vi "Check parts acceptable - baselayer.vi"(8 "error in (no error)":errorcluster, 9 "Baselayer IDs":string[](array[string]), 10 "DB out base":string[][](array[string]), 11 "Database Entry in":refnum<class "Database Entry.lvclass">) -> (0 "error out":errorcluster, 1 "Thickness out":string[](array[string]), 2 "Replace parts out":bool, 3 "Database Entry out":refnum<class "Database Entry.lvclass">, 4 "Abort?":bool)   [LabVIEW 2021, in "Database Entry.lvclass"]
uses:
  Database Entry.lvclass
  Database Entry.lvclass/Database Entry.ctl
  Components/Stack/Stack.lvclass
panel:
  in  "Replace parts base":bool
  in  "Thickness column options to use for assembly":u16(ring) items=["avg_thickness", "max_thickness"]
  in  "Are these parts satisfactory?":bool
  in  "Abort":bool
  in  "Submit":bool
  in  "Proposed thickness for assembly dispense":string[](array[string])
  in  "Database out - baselayer":i32[](listbox)
  # "Modify thickness values manually, if needed"
  # "(If parts are satisfactory, this assembly run will be written into Postgres.)"
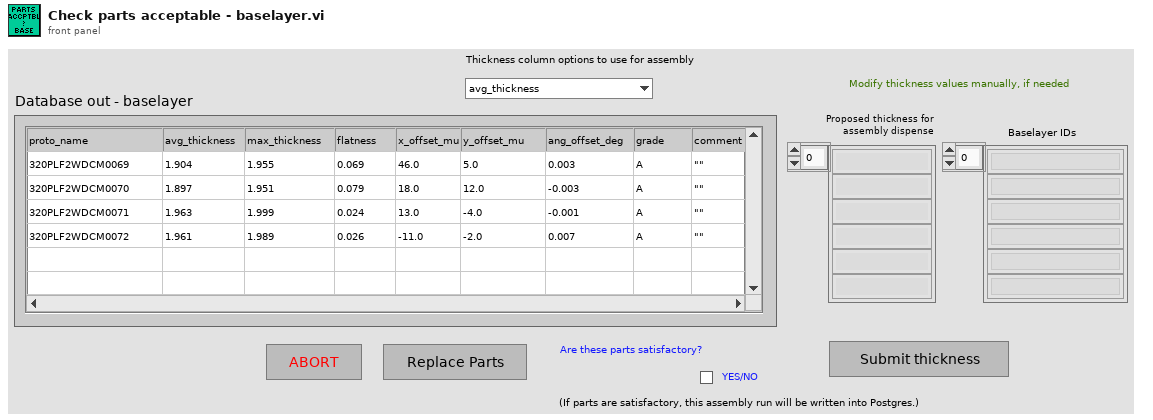
[diagram p1: front panel]
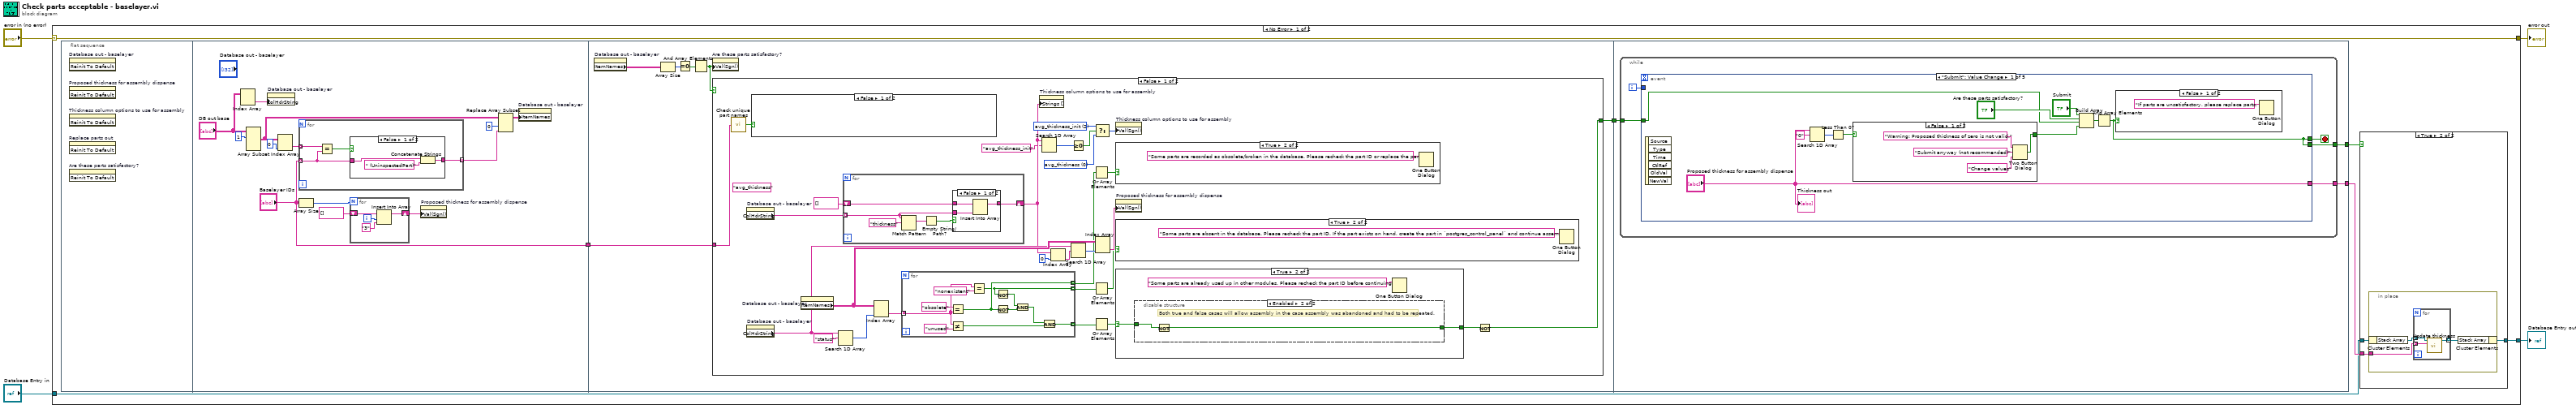
[diagram p0: block diagram]
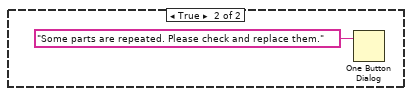
[diagram p5: hidden frame]
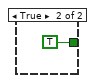
[diagram p10: hidden frame]
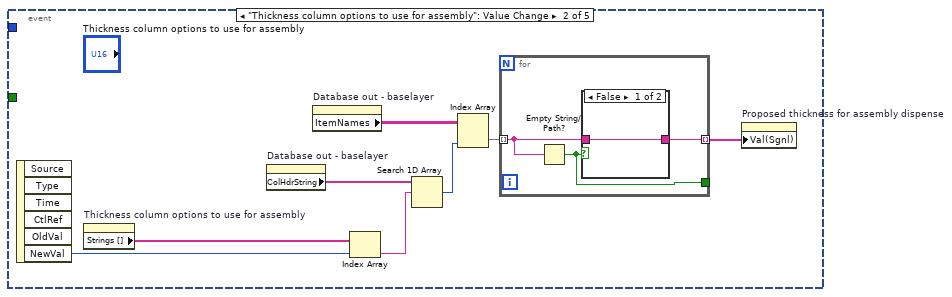
[diagram p13: hidden frame]
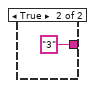
[diagram p14: hidden frame]
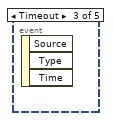
[diagram p15: hidden frame]
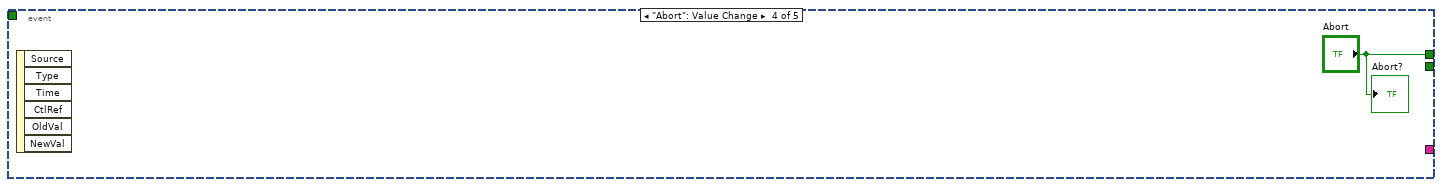
[diagram p16: hidden frame]
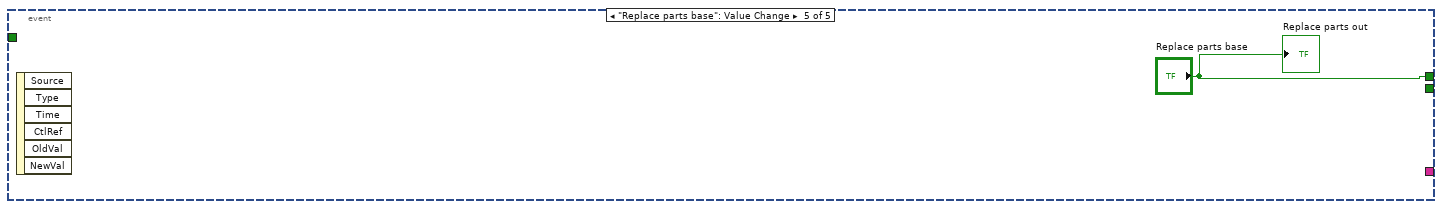
[diagram p17: hidden frame]
diagram:
  n1 = case shown="No Error" "error in (no error)" {
    selector: "error in (no error)" -> [w11 w153]
    tunnel: [w11 w153] -> w3
    tunnel: [w7 w152] -> w1
    tunnel: "Database Entry in" -> [w8 w152]
    frame No Error {
      n2 = flat-sequence {
        tunnel: ["Baselayer IDs"] -> w6
        tunnel: w6 -> [w47]
        tunnel: [w48] -> w5
        tunnel: [w115] -> w10
        tunnel: [w114] -> w9
        tunnel: w5 -> [w113]
        frame #0 {
          n3 = invoke on="Database out - baselayer" class="MCListbox (strict)" method="Reinit To Default"() -> ()  [unwired: 3 in, 3 out]
          n4 = invoke on="Proposed thickness for assembly dispense" class="Arr (strict)" method="Reinit To Default"() -> ()  [unwired: 3 in, 3 out]
          n5 = invoke on="Thickness column options to use for assembly" class="Ring (strict)" method="Reinit To Default"() -> ()  [unwired: 3 in, 3 out]
          n6 = invoke on="Replace parts out" class="Bool (strict)" method="Reinit To Default"() -> ()  [unwired: 3 in, 3 out]
          n7 = invoke on="Are these parts satisfactory?" class="Bool (strict)" method="Reinit To Default"() -> ()  [unwired: 3 in, 3 out]
        }
        frame #1 {
          n8 = Index Array(array="DB out base") -> (element=w27:string[])  [unwired: 2 in]
          n9 = Array Subset(array="DB out base", index (row)=1 ("index")) -> (w31:string[][])  [unwired: 3 in]
          n10 = property on="Database out - baselayer" class="MCListbox (strict)"("ColHdrString"=w27) -> ()  [unwired: 2 in, 2 out]
          n11 = Index Array(array=w31, index (col)=0 ("disabled index (col)")) -> (element=w32:string[])  [unwired: 1 in]
          n12 = for {
            tunnel: w32 -> [w41] mode=indexing
            tunnel: "Baselayer IDs" -> [w39] mode=indexing
            tunnel: [w40] -> w29 mode=indexing
            n13 = Equal?(x=w41, y=w39) -> (x = y?=w42:bool)
            n14 = case shown="False" w42 {
              tunnel: w39 -> [w45 w46]
              tunnel: [w43 w46] -> w40
              frame False {
                n15 = Concatenate Strings(w45, " (UninspectedPart)" ("string")) -> (w43:string)
              }
              frame True {
              }
            }
          }
          n16 = Array Size(array="Baselayer IDs") -> (size(s)=w25:i32)
          n17 = for {
            N: w25 -> [_]
            shift-right: [w35] -> w23
            shift-left: string[] [] -> [w38]
            i -> [w36]
            n18 = Insert Into Array(array=w38, index=w36, new element="3" ("new element/subarray")) -> (w35:string[])
          }
          n19 = property on="Proposed thickness for assembly dispense" class="Arr (strict)"("Val(Sgnl)"=w23) -> ()  [unwired: 2 in, 2 out]
          n20 = Replace Array Subset(array=w31, new element=w29, index (col)=0 ("disabled index (col)")) -> (w26:string[][])  [unwired: 1 in]
          n21 = property on="Database out - baselayer" class="MCListbox (strict)"("ItemNames"=w26) -> ()  [unwired: 2 in, 2 out]
        }
        frame #2 {
          n22 = property on="Database out - baselayer" class="MCListbox (strict)"() -> ("ItemNames"=w50:string[][])  [unwired: 2 in, 2 out]
          n23 = Array Size(array=w50) -> (size(s)=w51:i32[])
          n24 = Equal To 0?(x=w51) -> (x = 0?=w52:bool[])
          n25 = And Array Elements(Boolean array=w52) -> (logical AND=w49:bool)
          n26 = property on="Are these parts satisfactory?" class="Bool (strict)"("Val(Sgnl)"=w49) -> ()  [unwired: 2 in, 2 out]
          n27 = case shown="False" w49 {
            tunnel: w47 -> [w69 _]
            tunnel: [w66 TRUE] -> w48
            frame False {
              w53 = u16 0 items=["avg_thickness", "max_thickness", "avg_thickness_init", "max_thickness_init"] ("Thickness column options to use for assembly")
              w55 = u16 2 items=["avg_thickness", "max_thickness", "avg_thickness_init", "max_thickness_init"] ("Thickness column options to use for assembly")
              (unwired) "avg_thickness" ("f")
              n28 = call "Check unique part names.vi"("Part IDs"=w69) -> ("Parts repeated"=w68:bool)
              n29 = property on="Database out - baselayer" class="MCListbox (strict)"() -> ("ColHdrString"=w79:string[])  [unwired: 2 in, 2 out]
              n30 = property on="Database out - baselayer" class="MCListbox (strict)"() -> ("ColHdrString"=w73:string[])  [unwired: 2 in, 2 out]
              n31 = case shown="False" w68 {
                frame False {
                }
                frame True {
                  n32 = One Button Dialog(message="Some parts are repeated. Please check and replace them.") -> ()  [unwired: 1 in, 1 out]
                }
              }
              n33 = property on="Database out - baselayer" class="MCListbox (strict)"() -> ("ItemNames"=w74:string[][])  [unwired: 2 in, 2 out]
              n34 = Search 1D Array(1D array=w73, element="status") -> (index of element=w71:i32)  [unwired: 1 in]
              n35 = for {
                tunnel: w79 -> [w104] mode=indexing
                shift-right: [w103] -> w59
                shift-left: string[] [] -> [w102]
                n36 = Match Pattern(string=w104, regular expression="thickness") -> (match substring=w106:string)  [unwired: 1 in, 3 out]
                n37 = Empty String/Path?(string/path=w106) -> (empty?=w105:bool)
                n38 = case shown="False" w105 {
                  tunnel: [w108 w111] -> w103
                  tunnel: w104 -> [w109 _]
                  tunnel: w102 -> [w110 w111]
                  frame False {
                    n39 = Insert Into Array(array=w110, new element=w109) -> (w108:string[])  [unwired: 1 in]
                  }
                  frame True {
                  }
                }
              }
              n40 = Index Array(array=w74, index (col)=w71) -> (element=w65:string[])  [unwired: 1 in]
              n41 = for {
                tunnel: w65 -> [w91] mode=indexing
                tunnel: [w98] -> w63 mode=indexing
                tunnel: [w95] -> w64 mode=indexing
                tunnel: [w97] -> w61 mode=indexing
                n42 = Equal?(x="obsolete" ("y"), y=w91) -> (x = y?=w97:bool)
                n43 = Not Equal?(x=w91, y="unused") -> (x != y?=w100:bool)
                n44 = Equal?(x=w91, y="nonexistent") -> (x = y?=w95:bool)
                n45 = Not(x=w95) -> (.not. x?=w94:bool)
                n46 = Not(x=w97) -> (.not. x?=w96:bool)
                n47 = And(x=w94, y=w96) -> (x .and. y?=w93:bool)
                n48 = And(x=w93, y=w100) -> (x .and. y?=w98:bool)
              }
              n49 = property on="Thickness column options to use for assembly" class="Ring (strict)"("Strings []"=w59) -> ()  [unwired: 2 in, 2 out]
              n50 = Search 1D Array(1D array=w59, element="avg_thickness_init") -> (index of element=w58:i32)  [unwired: 1 in]
              n51 = Index Array(array=w59, index=0) -> (element=w80:string)
              n52 = Greater Or Equal To 0?(x=w58) -> (x >= 0?=w57:bool)
              n53 = Search 1D Array(1D array=w73, element=w80) -> (index of element=w76:i32)  [unwired: 1 in]
              n54 = Or Array Elements(Boolean array=w61) -> (logical OR=w60:bool)
              n55 = Or Array Elements(Boolean array=w64) -> (logical OR=w70:bool)
              n56 = Or Array Elements(Boolean array=w63) -> (logical OR=w62:bool)
              n57 = Select(t=w55, s=w57, f=w53) -> (s? t:f=w54:u16)
              n58 = Index Array(array=w74, index (col)=w76) -> (element=w75:string[])  [unwired: 1 in]
              n59 = property on="Thickness column options to use for assembly" class="Ring (strict)"("Val(Sgnl)"=w54) -> ()  [unwired: 2 in, 2 out]
              n60 = case shown="True" w60 {
                frame False {
                }
                frame True {
                  n61 = One Button Dialog(message="Some parts are recorded as obsolete/broken in the database. Please recheck the part ID or replace the part.") -> ()  [unwired: 1 in, 1 out]
                }
              }
              n62 = property on="Proposed thickness for assembly dispense" class="Arr (strict)"("Val(Sgnl)"=w75) -> ()  [unwired: 2 in, 2 out]
              n63 = case shown="True" w70 {
                frame False {
                }
                frame True {
                  n64 = One Button Dialog(message="Some parts are absent in the database. Please recheck the part ID. If the part exists on hand, create the part in `postgres_control_panel` and continue assembly. ") -> ()  [unwired: 1 in, 1 out]
                }
              }
              n65 = case shown="True" w62 {
                selector: w62 -> [w83 w85]
                tunnel: [w83 w84] -> w67
                frame False {
                }
                frame True {
                  n66 = disable-structure shown="Enabled" {
                    disable-tunnel: w85 -> [w87 w89]
                    disable-tunnel: [w87 w88] -> w84
                    frame Disabled {
                    }
                    frame Enabled {
                      # "Both true and false cases will allow assembly in the case assembly was abandoned and had to be repeated."
                      n67 = Not(x=w89) -> (.not. x?=w88:bool)
                    }
                  }
                  n68 = One Button Dialog(message="Some parts are already used up in other modules. Please recheck the part ID before continuing.") -> ()  [unwired: 1 in, 1 out]
                }
              }
              n69 = Not(x=w67) -> (.not. x?=w66:bool)
            }
            frame True {
            }
          }
        }
        frame #3 {
          n70 = while {
            tunnel: [w118] -> w115
            tunnel: [w120] -> w114
            tunnel: w113 -> [w117]
            i -> [w116]
            stop <- w119 stop-if-true
            n71 = event shown="[0] \"Submit\": Value Change" {
              selector: _ -> [_ _ _ _ _]
              dyn-events: _ -> [_ _ _ _ _]
              timeout: _ -> [_ _ _ _ _]
              tunnel: [w126 _ _ "Abort" "Replace parts base"] -> w119
              tunnel: ["Proposed thickness for assembly dispense" _ _ _ _] -> w120
              tunnel: [w126 _ _ _ _] -> w118
              tunnel: w117 -> [w127 _ _ _ _]
              tunnel: w116 -> [_ _ _ _ _]
              event "Submit": Value Change {
                n72 = event-data() -> ()  [unwired: 1 in, 6 out]
                n73 = Search 1D Array(1D array="Proposed thickness for assembly dispense", element="0") -> (index of element=w123:i32)  [unwired: 1 in]
                n74 = Less Than 0?(x=w123) -> (x < 0?=w122:bool)
                n75 = case shown="False" w122 {
                  selector: w122 -> [_ w135]
                  tunnel: [w134 w135] -> w121
                  frame False {
                    n76 = Two Button Dialog(message="Warning: Proposed thickness of zero is not valid.", 1:"Change values" ("T button name (\"OK\")"), 2:"Submit anyway (not recommended)" ("F button name (\"Cancel\")")) -> (T button?=w134:bool)
                  }
                  frame True {
                  }
                }
                n77 = Build Array("Submit", "Are these parts satisfactory?", w127, w121) -> (w130:bool[])
                n78 = And Array Elements(Boolean array=w130) -> (logical AND=w126:bool)
                n79 = case shown="False" w126 {
                  frame False {
                    n80 = One Button Dialog(message="If parts are unsatisfactory, please replace parts. ") -> ()  [unwired: 1 in, 1 out]
                  }
                  frame True {
                  }
                }
                "Thickness out" <- "Proposed thickness for assembly dispense"
              }
              event "Thickness column options to use for assembly": Value Change {
                n81 = event-data() -> ("NewVal"=w143:u16)  [unwired: 1 in, 5 out]
                n82 = property on="Thickness column options to use for assembly" class="Ring (strict)"() -> ("Strings []"=w144:string[])  [unwired: 2 in, 2 out]
                n83 = property on="Database out - baselayer" class="MCListbox (strict)"() -> ("ColHdrString"=w140:string[])  [unwired: 2 in, 2 out]
                n84 = property on="Database out - baselayer" class="MCListbox (strict)"() -> ("ItemNames"=w141:string[][])  [unwired: 2 in, 2 out]
                n85 = Index Array(array=w144, index=w143) -> (element=w142:string)
                n86 = Search 1D Array(1D array=w140, element=w142) -> (index of element=w139:i32)  [unwired: 1 in]
                n87 = Index Array(array=w141, index (col)=w139) -> (element=w138:string[])  [unwired: 1 in]
                n88 = for {
                  tunnel: w138 -> [w147] mode=indexing
                  tunnel: [w146] -> w137 mode=indexing
                  tunnel: [w145] -> _
                  n89 = Empty String/Path?(string/path=w147) -> (empty?=w145:bool)
                  n90 = case shown="False" w145 {
                    tunnel: w147 -> [w148 _]
                    tunnel: [w148 "3"] -> w146
                    frame False {
                    }
                    frame True {
                    }
                  }
                }
                n91 = property on="Proposed thickness for assembly dispense" class="Arr (strict)"("Val(Sgnl)"=w137) -> ()  [unwired: 2 in, 2 out]
              }
              event Timeout {
                n92 = event-data() -> ()  [unwired: 1 in, 3 out]
              }
              event "Abort": Value Change {
                n93 = event-data() -> ()  [unwired: 1 in, 6 out]
                "Abort?" <- "Abort"
              }
              event "Replace parts base": Value Change {
                n94 = event-data() -> ()  [unwired: 1 in, 6 out]
                "Replace parts out" <- "Replace parts base"
              }
            }
          }
        }
      }
      n95 = case shown="True" w10 {
        tunnel: [w12 w15] -> w7
        tunnel: w8 -> [w12 w13]
        tunnel: w9 -> [_ w14]
        frame False {
        }
        frame True {
          n96 = in-place {
            in-place-border: w14 -> [w16]
            n97 = in-place-cluster #1(w13) -> ("Stack Array"=w18:refnum<class "Stack.lvclass">[])
            n98 = for {
              tunnel: w18 -> [w20] mode=indexing
              tunnel: [w19] -> w17 mode=indexing
              tunnel: w16 -> [w21] mode=indexing
              n99 = call "Update thickness.vi"("Thickness"=w21, "Stack in"=w20) -> ("Stack out"=w19:refnum<class "Stack.lvclass">)  [unwired: 8 in, 1 out]
            }
            n100 = in-place-cluster #1("Stack Array"=w17) -> (w15:refnum<class "Database Entry.lvclass">)
          }
        }
      }
    }
    frame Error {
    }
  }
  "error out" <- w3
  "Database Entry out" <- w1
